vi "from_string.vi"(5 "type":refnum<class "Bytes.lvclass">, 11 "string_data":T1) -> (3 "Bytes out":refnum<class "Bytes.lvclass">)   [LabVIEW 2020, in "variant.lvlib" / "Bytes.lvclass"]
uses:
  Bytes.lvclass
  data.ctl
  Bytes.lvclass/Bytes.ctl
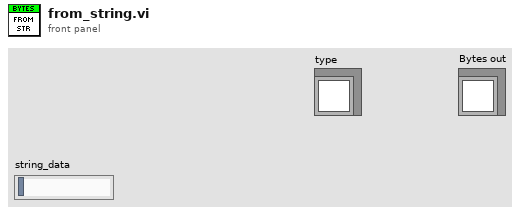
[diagram p1: front panel]
types:
  T1 = typedef "variant.lvlib/Bytes.lvclass/data.ctl" = string
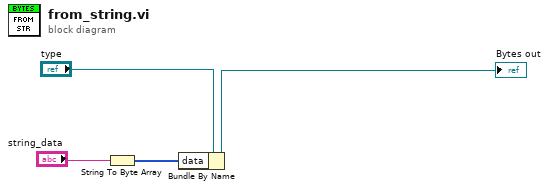
[diagram p0: block diagram]
diagram:
  n1 = String To Byte Array(string="string_data") -> (unsigned byte array=w1:u8[])
  n2 = Bundle By Name(cluster="type", "data"=w1) -> (→"Bytes out":refnum<class "Bytes.lvclass">)
